vi "SPI FPGA.vi"   [LabVIEW 2014]
uses:
  SPIBus0/IO Node Logic Template_SPIBus0.lvlib
  <vilib>/rvi/DataTransferAndStorage/Container/XNode/niFpgaContainer.xnode
  <vilib>/rvi/interface/RandomDataEmulation/nirviRandomDataFpgaReadWriteTemplate.vi
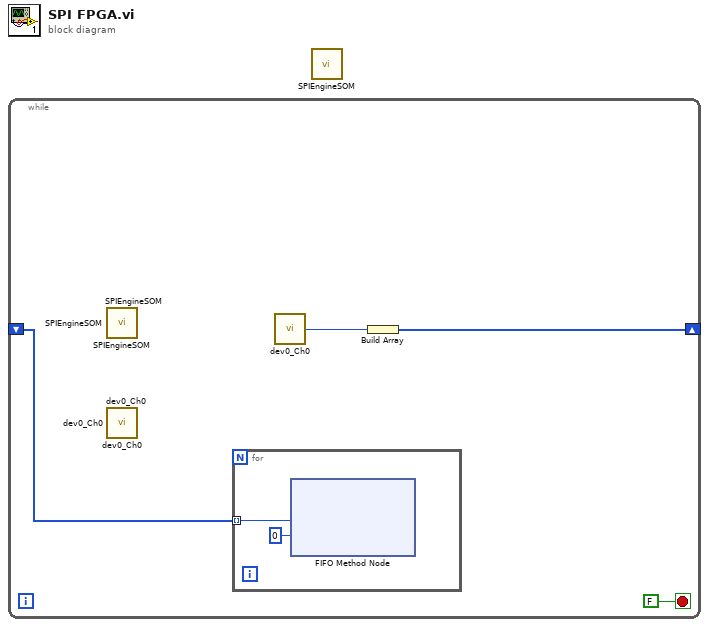
[diagram p0: block diagram]
diagram:
  n1 = while {
    shift-right: [w4] -> _
    shift-left: _ -> [w3]
    stop <- FALSE stop-if-true
    n2 = for {
      tunnel: w3 -> [w6] mode=indexing
      n3 = xnode ("FIFO Method Node")("Element"=w6, "Timeout"=0) -> ()  [unwired: 1 in, 2 out]
    }
    n4 = call "dev0_Ch0.vi"() -> ("Received Data"=w1:u64)  [unwired: 15 in]
    n5 = Build Array(w1) -> (w4:u64[])
  }
  n6 = call "SPIEngineSOM.vi"() -> ()  [unwired: 12 in]
  n7 = call "SPIEngineSOM.vi"() -> ()  [unwired: 12 in]
  n8 = call "SPIEngineSOM.vi"() -> ()  [unwired: 12 in]
  n9 = call "dev0_Ch0.vi"() -> ()  [unwired: 15 in, 1 out]
  n10 = call "dev0_Ch0.vi"() -> ()  [unwired: 15 in, 1 out]
  n11 = call "dev0_Ch0.vi"() -> ()  [unwired: 15 in, 1 out]
  n12 = call "SPIEngineSOM.vi"() -> ()  [unwired: 12 in]
